vi "GetXL_CellValues_2D_Dbl.vi"(8 "error in (no error)":errorcluster, 9 "End":cluster{"Column":i32, "Row":i32}, 10 "Start":cluster{"Column":i32, "Row":i32}, 11 "Refnum Cluster In":T1) -> (0 "error out":errorcluster, 2 "data":dbl[][](array[numeric]), 3 "Refnum Cluster Out":T1)   [LabVIEW 2017, in "excel_configuration.lvlib"]
doc: "Reads the range between Start and End from the open worksheet as a two-dimensional array of doubles."
uses:
  excel_configuration.lvlib
  d7ffd489-c8e5-4946-98fc-02ab110a5fd3.vi
  <vilib>/Utility/error.llb/Clear Errors.vi
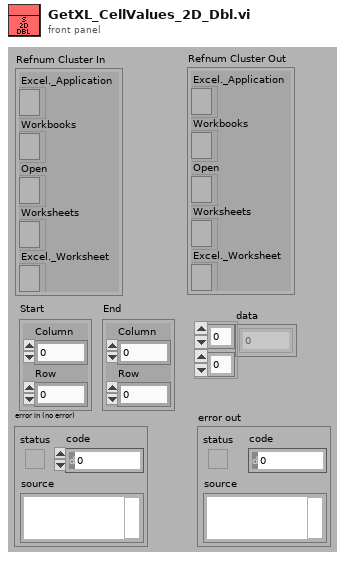
[diagram p1: front panel]
types:
  T1 = cluster{"Excel._Application":refnum<k7>, "Workbooks":refnum<k7>, "Open":refnum<k7>, "Worksheets":refnum<k7>, "Excel._Worksheet":refnum<k7>}
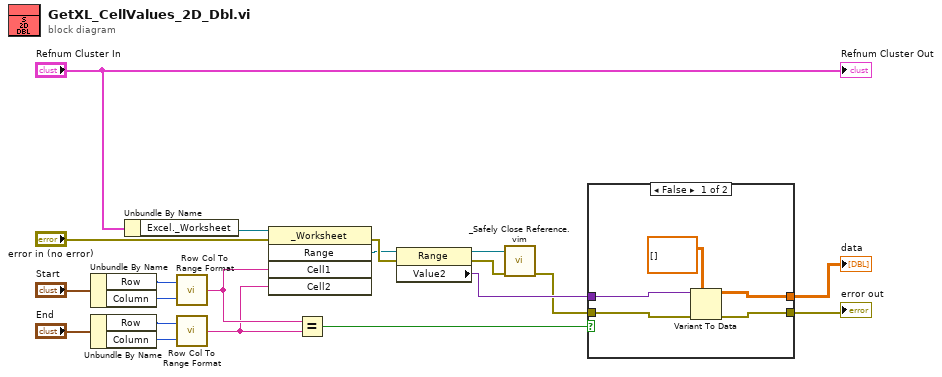
[diagram p0: block diagram]
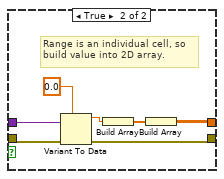
[diagram p2: hidden frame]
diagram:
  n1 = Unbundle By Name("Start") -> ("Row"=w14:i32, "Column"=w13:i32)
  n2 = Unbundle By Name("End") -> ("Row"=w11:i32, "Column"=w10:i32)
  n3 = Unbundle By Name("Refnum Cluster In") -> ("Excel._Worksheet"=w2:refnum<k7>)
  n4 = call "Row Col To Range Format.vi"("Column"=w13, "Row"=w14) -> ("Output String"=w5:string)
  n5 = call "Row Col To Range Format.vi"("Column"=w10, "Row"=w11) -> ("Output String"=w4:string)
  n6 = invoke class="_Worksheet" method="Range"(reference=w2, error in="error in (no error)", "Cell1"=w5, "Cell2"=w4) -> (error out=w19:errorcluster, "Range"=w18:refnum<k7>)  [unwired: 1 in, 3 out]
  n7 = Equal?(x=w5, y=w4) -> (x = y?=w3:bool)
  n8 = property class="Range"(reference=w18, error in=w19) -> (reference out=w17:refnum<k7>, error out=w16:errorcluster, "Value2"=w9:variant)
  n9 = call "_Safely Close Reference.vim"("error in (no error)"=w16, "Automation Refnum in"=w17) -> ("error out"=w8:errorcluster)  [unwired: 9 in]
  n10 = case shown="False" w3 {
    tunnel: w9 -> [w25 w32]
    tunnel: [w23 w27] -> w6
    tunnel: [w22 w26] -> w7
    tunnel: w8 -> [w21 w31]
    frame False {
      n11 = Variant To Data(error in=w21, type=dbl[][] [], Variant=w25) -> (data=w23:dbl[][], error out=w22:errorcluster)
    }
    frame True {
      # "Range is an individual cell, so\nbuild value into 2D array."
      n12 = Variant To Data(error in=w31, type=0.0, Variant=w32) -> (data=w29:dbl, error out=w26:errorcluster)
      n13 = Build Array(w29) -> (w28:dbl[])
      n14 = Build Array(w28) -> (w27:dbl[][])
    }
  }
  "error out" <- w7
  "data" <- w6
  "Refnum Cluster Out" <- "Refnum Cluster In"
